vi "SaveUISettings.vi"(8 "Error In":errorcluster, 11 "UI References":T1) -> (0 "Error Out":errorcluster)   [LabVIEW 2017, in "Client.lvlib" / "UI_API.lvlib"]
uses:
  UI_API.lvlib
  TypeDefs/UIReferences.ctl
  <vilib>/Utility/miscctls.llb/LVRowAndColumnTypeDef.ctl
  <vilib>/Utility/config.llb/Write Key (I32).vi
  <vilib>/Utility/config.llb/Write Key (String).vi
  <vilib>/Utility/config.llb/Write Key (Boolean).vi
  <vilib>/Utility/config.llb/NI_LVConfig.lvlib
  Client.lvlib
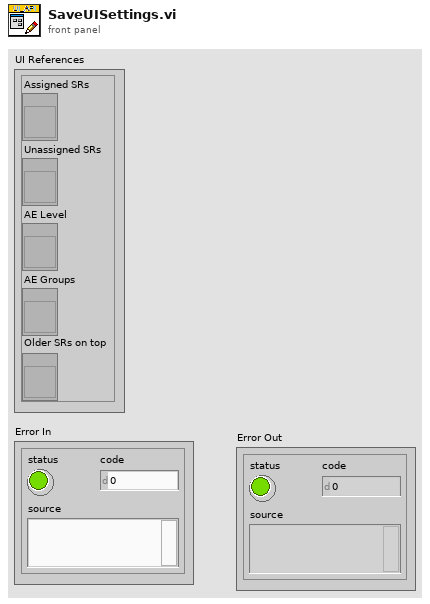
[diagram p1: front panel]
types:
  T1 = typedef "Client.lvlib/UI_API.lvlib/UIReferences.ctl" = cluster{"Assigned SRs":refnum<vi>, "Unassigned SRs":refnum<vi>, "AE Level":refnum<vi>, "AE Groups":refnum<vi>, "Older SRs on top":refnum<vi>}
  T2 = typedef "LVRowAndColumnTypeDef.ctl" = cluster{"Row":i32, "Column":i32}
  T3 = typedef "NI_LVConfig.lvlib/Config Data RefNum.ctl" = refnum<k1>
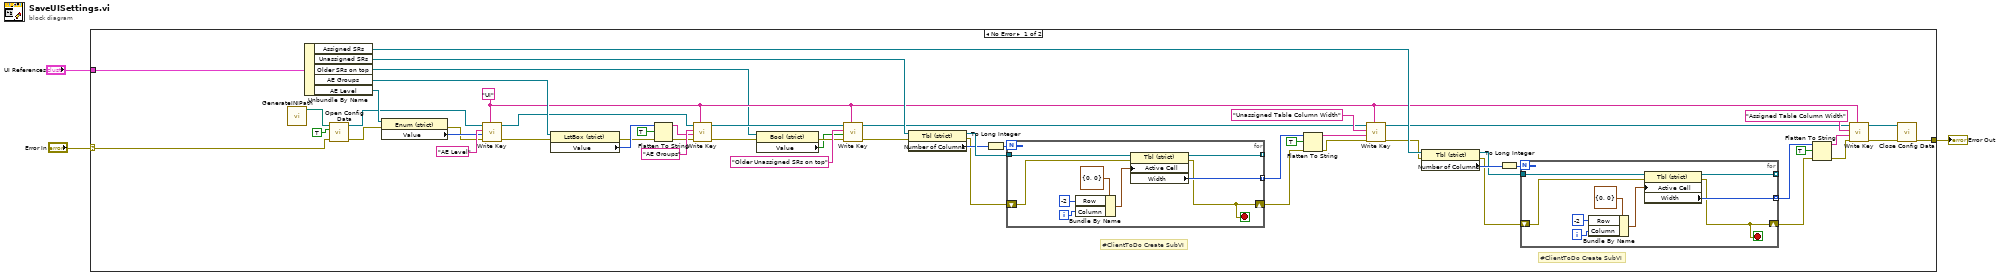
[diagram p0: block diagram]
diagram:
  n1 = case shown="No Error" "Error In" {
    selector: "Error In" -> [w57 w77]
    tunnel: "UI References" -> [w56 _]
    tunnel: [w40 w77] -> w1
    frame No Error {
      w9 = "UI" ("section")
      # "#ClientToDo Create SubVI"
      # "#ClientToDo Create SubVI"
      n2 = call "GenerateINIPath.vi"() -> ("INI Path"=w13:path)  [unwired: 11 in]
      n3 = Unbundle By Name(w56) -> ("Assigned SRs"=w27:refnum<vi>, "Unassigned SRs"=w39:refnum<vi>, "Older SRs on top"=w7:refnum<vi>, "AE Groups"=w48:refnum<vi>, "AE Level"=w54:refnum<vi>)
      n4 = call <vilib>:"Open Config Data.vi"("error in (no error)"=w57, "create file if necessary (T)"=TRUE ("create file if necessary? (T)"), "configuration file path"=w13) -> ("error out"=w52:errorcluster, "refnum"=w50:T3)  [unwired: 6 in, 1 out]
      n5 = property class="Enum (strict)"(reference=w54, error in=w52) -> (error out=w51:errorcluster, "Value"=w53:enum16{"AE / ELP", "AE Intern"})  [unwired: 1 out]
      n6 = call-poly <vilib>:"Write Key.vi"("section"=w9, "error in (no error)"=w51, "value"=w53, "key"="AE Level", "refnum"=w50) -> ("error out"=w47:errorcluster, "refnum out"=w41:T3)  [unwired: 4 in, 1 out]
      n7 = property class="LstBox (strict)"(reference=w48, error in=w47) -> (error out=w43:errorcluster, "Value"=w46:i32[])  [unwired: 1 out]
      n8 = Flatten To String(anything=w46, prepend array or string size? (T)=TRUE, error in (no error)=w43) -> (data string=w44:string, error out=w42:errorcluster)  [unwired: 1 in, 1 out]
      n9 = call-poly <vilib>:"Write Key.vi"("section"=w9, "error in (no error)"=w42, "value"=w44, "key"="AE Groups", "refnum"=w41) -> ("error out"=w6:errorcluster, "refnum out"=w11:T3)  [unwired: 4 in, 1 out]
      n10 = property class="Bool (strict)"(reference=w7, error in=w6) -> (error out=w5:errorcluster, "Value"=w4:bool)  [unwired: 1 out]
      n11 = call-poly <vilib>:"Write Key.vi"("section"=w9, "error in (no error)"=w5, "value"=w4, "key"="Older Unassigned SRs on top", "refnum"=w11) -> ("error out"=w12:errorcluster, "refnum out"=w10:T3)  [unwired: 4 in, 1 out]
      n12 = property class="Tbl (strict)"(reference=w39, error in=w12) -> (reference out=w38:refnum<vi>, error out=w25:errorcluster, "Number of Columns"=w37:u32)
      n13 = To Long Integer(number=w37) -> (32bit integer=w36:i32)
      n14 = for {
        N: w36 -> [_]
        shift-right: [w69] -> w26
        shift-left: w25 -> [w70]
        tunnel: w38 -> [w76]
        tunnel: [w72] -> w34 mode=indexing
        tunnel: [w71] -> _ mode=indexing
        i -> [w68]
        stop <- w69 stop-if-true
        n15 = Bundle By Name(cluster=T2 {"Row"=0, "Column"=0} ("Active Cell:Active Cell"), "Row"=-2, "Column"=w68) -> (w73:T2)
        n16 = property class="Tbl (strict)"(reference=w76, error in=w70, "Active Cell"=w73) -> (reference out=w71:refnum<vi>, error out=w69:errorcluster, "Width"=w72:u32)
      }
      n17 = Flatten To String(anything=w34, prepend array or string size? (T)=TRUE, error in (no error)=w26) -> (data string=w32:string, error out=w33:errorcluster)  [unwired: 1 in, 1 out]
      n18 = call-poly <vilib>:"Write Key.vi"("section"=w9, "error in (no error)"=w33, "value"=w32, "key"="Unassigned Table Column Width", "refnum"=w10) -> ("error out"=w22:errorcluster, "refnum out"=w20:T3)  [unwired: 4 in, 1 out]
      n19 = property class="Tbl (strict)"(reference=w27, error in=w22) -> (reference out=w28:refnum<vi>, error out=w24:errorcluster, "Number of Columns"=w29:u32)
      n20 = To Long Integer(number=w29) -> (32bit integer=w30:i32)
      n21 = for {
        N: w30 -> [_]
        shift-right: [w60] -> w17
        shift-left: w24 -> [w61]
        tunnel: w28 -> [w67]
        tunnel: [w63] -> w16 mode=indexing
        tunnel: [w62] -> _ mode=indexing
        i -> [w59]
        stop <- w60 stop-if-true
        n22 = Bundle By Name(cluster=T2 {"Row"=0, "Column"=0} ("Active Cell:Active Cell"), "Row"=-2, "Column"=w59) -> (w64:T2)
        n23 = property class="Tbl (strict)"(reference=w67, error in=w61, "Active Cell"=w64) -> (reference out=w62:refnum<vi>, error out=w60:errorcluster, "Width"=w63:u32)
      }
      n24 = Flatten To String(anything=w16, prepend array or string size? (T)=TRUE, error in (no error)=w17) -> (data string=w14:string, error out=w15:errorcluster)  [unwired: 1 in, 1 out]
      n25 = call-poly <vilib>:"Write Key.vi"("section"=w9, "error in (no error)"=w15, "value"=w14, "key"="Assigned Table Column Width", "refnum"=w20) -> ("error out"=w21:errorcluster, "refnum out"=w19:T3)  [unwired: 4 in, 1 out]
      n26 = call <vilib>:"Close Config Data.vi"("error in (no error)"=w21, "refnum"=w19) -> ("error out"=w40:errorcluster)  [unwired: 8 in, 1 out]
    }
    frame Error {
    }
  }
  "Error Out" <- w1
